vi "RSZVB Trace Export Data With Options Extended.vi"(4 "Export Format (0: Unformatted)":i32(ring) items=["Unformatted", "Formatted"], 5 "Field Separator (0: Semicolon)":i32(ring) items=["Semicolon", "Comma", "Tabulator", "Space"], 6 "Decimal Separator (0: Point)":i32(ring) items=["Point", "Comma"], 7 "Export Data (0: Complex Values)":i32(ring) items=["Complex Values", "Linear magnitude and phase", "dB-magnitude and phase"], 8 "error in (no error)":errorcluster {"code" format="%.0x"}, 9 "File Name (Trc1.s1p)":string="Trc1.s1p", 10 "Trace Name (Trc1)":string="Trc1", 11 "VISA session":refnum<visa-resource-name>) -> (0 "error out":errorcluster {"code" format="%.0x"}, 3 "dup VISA session":refnum<visa-resource-name>)   [LabVIEW 2011]
doc: "This VI stores the trace data of a specified trace to a trace file.\n\nNote(s):\n\nTraces are created using the CALCulte<Ch>:PARameter:SDEFine... command.\n\n*.s<n>p touchstone files (<n> = 2, 3, 4) are intended for a complete set of <n>-port S-parameters. Data export fails if the active channel does not contain the full set of <n>^2 traces. If the necessary trace are available, '<trc_name>' can be the name of any of the traces.\n\nRemote-control command(s):\nMMEMory:STORe:TRACe '<trc_name>','<file_name>'[,UNFormatted | FORMatted, COMPlex | LINPhase | LOGPhase, POINt | COMMa, SEMicolon | COMMa | TABulator | SPACe]"
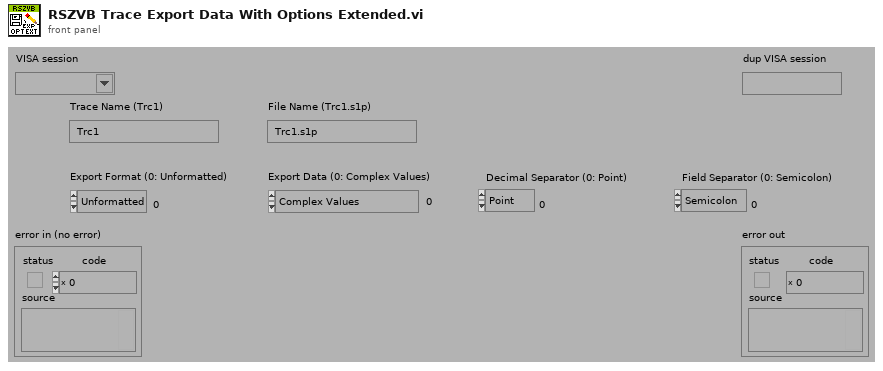
[diagram p1: front panel]
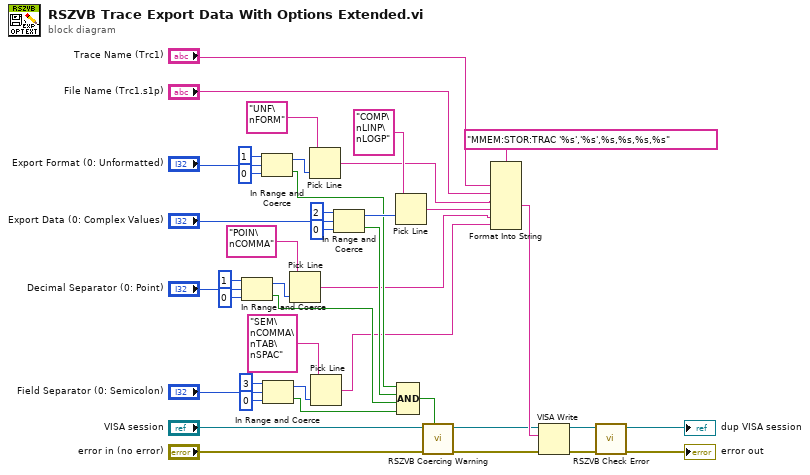
[diagram p0: block diagram]
diagram:
  n1 = In Range and Coerce(upper limit=1, x="Decimal Separator (0: Point)", lower limit=0) -> (coerced(x)=w11:i32, In Range?=w8:bool)
  n2 = In Range and Coerce(upper limit=1, x="Export Format (0: Unformatted)", lower limit=0) -> (coerced(x)=w29:i32, In Range?=w25:bool)
  n3 = In Range and Coerce(upper limit=3, x="Field Separator (0: Semicolon)", lower limit=0) -> (coerced(x)=w4:i32, In Range?=w2:bool)
  n4 = Pick Line(multi-line string="POIN\nCOMMA", line index=w11) -> (output string=w9:string)  [unwired: 1 in]
  n5 = Pick Line(multi-line string="UNF\nFORM", line index=w29) -> (output string=w34:string)  [unwired: 1 in]
  n6 = Pick Line(multi-line string="SEM\nCOMMA\nTAB\nSPAC", line index=w4) -> (output string=w1:string)  [unwired: 1 in]
  n7 = In Range and Coerce(upper limit=2, x="Export Data (0: Complex Values)", lower limit=0) -> (coerced(x)=w28:i32, In Range?=w26:bool)
  n8 = Pick Line(multi-line string="COMP\nLINP\nLOGP", line index=w28) -> (output string=w35:string)  [unwired: 1 in]
  n9 = Compound Arithmetic op=AND(w25, w26, w8, w2) -> (w27:bool)
  n10 = call "RSZVB Coercing Warning.vi"("In Range?"=w27, "error in (no error)"="error in (no error)", "VISA session"="VISA session") -> ("error out"=w23:errorcluster, "dup VISA session"=w24:refnum<visa-resource-name>)  [unwired: 7 in]
  n11 = Format Into String(format string="MMEM:STOR:TRAC '%s','%s',%s,%s,%s,%s", "Trace Name (Trc1)", "File Name (Trc1.s1p)", w34, w35, w9, w1) -> (resulting string=w38:string)  [unwired: 2 in, 1 out]
  n12 = VISA Write(VISA resource name=w24, write buffer=w38, error in (no error)=w23) -> (VISA resource name out=w39:refnum<visa-resource-name>, error out=w40:errorcluster)  [unwired: 1 out]
  n13 = call "RSZVB Check Error.vi"("error in (no error)"=w40, "VISA session"=w39) -> ("error out"=→"error out":errorcluster, "dup VISA session"=→"dup VISA session":refnum<visa-resource-name>)  [unwired: 8 in]
